vi "h.COMM.Write Command.vi"(6 "Request Option":T1, 8 "error in":errorcluster, 9 "Argument":string, 10 "Command":string, 11 "Connection ID":refnum<k5>) -> (0 "error out":errorcluster, 3 "Connection ID out":refnum<k5>)   [LabVIEW 2019, in "h.Library.lvlib"]
doc: "This vi sends a command and argument to a Hyperion instrument.\n\n<b>Connection ID</b> - is a network connection refnum that uniquely identifies the TCP connection\n<b>Command</b> - The command to execute\n<b>Request Options</b> - Option that controls how the command responds\n<b>error in</b> - describes error conditions that occur before this node runs. This input provides standard error functionality\n<b>Connection ID out</b> - Returns the same value as connection ID\n<b>error out</b> - contains error information. This output provides standard error out functionality."
uses:
  h.Library.lvlib
  CTL/h.COMM.RequestCommandOptions.ctl
panel:
  out "bytes written":i32
  # "Hyperion Write Command"
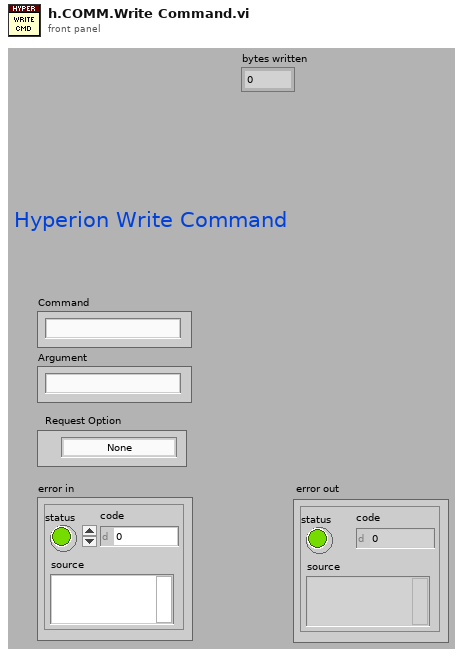
[diagram p1: front panel]
types:
  T1 = typedef "h.Library.lvlib/h.COMM.RequestCommandOptions.ctl" = enum8{"None", "Suppress Message", "Suppress Content", "Compress"}
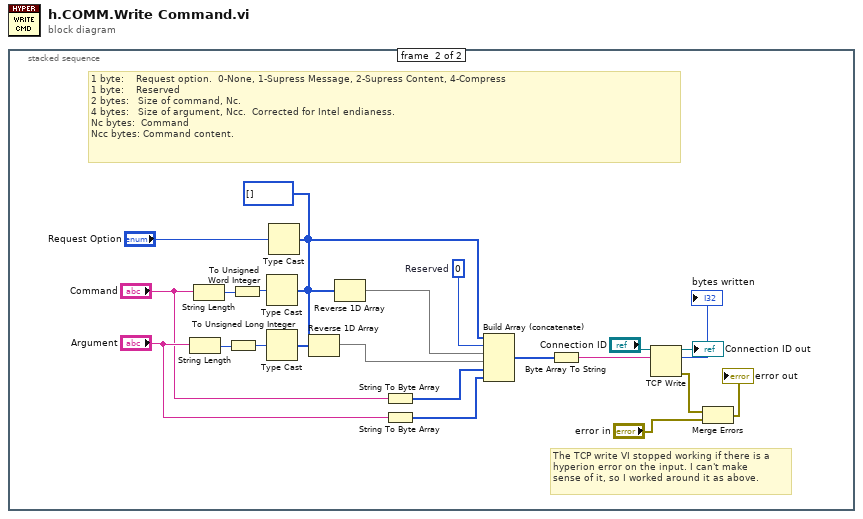
[diagram p0: block diagram]
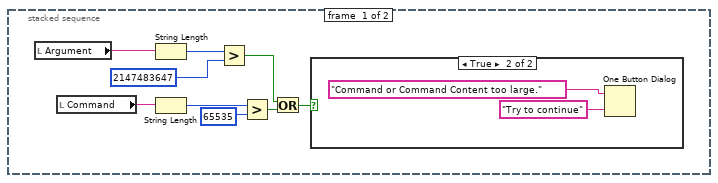
[diagram p2: hidden frame]
diagram:
  n1 = stacked-sequence {
    frame #0 {
      n2 = local read "Argument"() -> (w9:string)
      n3 = local read "Command"() -> (w8:string)
      n4 = String Length(string=w9) -> (length=w7:i32)
      n5 = String Length(string=w8) -> (length=w4:i32)
      n6 = Greater?(x=w7, y=2147483647) -> (0:w3:bool)
      n7 = Greater?(x=w4, y=65535) -> (0:w2:bool)
      n8 = Or(x=w3, y=w2) -> (x .or. y?=w1:bool)
      n9 = case shown="True" w1 {
        frame False {
        }
        frame True {
          n10 = One Button Dialog(message="Command or Command Content too large." ("[error source] (\" \")"), button name ("OK")="Try to continue") -> ()  [unwired: 1 out]
        }
      }
    }
    frame #1 {
      w22 = u8 0  # Reserved
      w16 = u8[] []
      # "The TCP write VI stopped working if there is a\nhyperion error on the input. I can't make\nsense of it, so I worked around it as above."
      # "1 byte:    Request option.  0-None, 1-Supress Message, 2-Supress Content, 4-Compress\n1 byte:    Reserved\n2 bytes:   Size of command, Nc.\n4 bytes:   Size of argument, Ncc.  Corrected for Intel endianess.\nNc bytes:  Command\nNcc bytes: Command content."
      n11 = String Length(string="Argument") -> (length=w32:i32)
      n12 = String Length(string="Command") -> (length=w33:i32)
      n13 = To Unsigned Long Integer(number=w32) -> (unsigned 32bit integer=w31:u32)
      n14 = To Unsigned Word Integer(number=w33) -> (unsigned 16bit integer=w21:u16)
      n15 = Type Cast(type=w16, x=w21) -> (*(type *) &x=w18:u8[])
      n16 = Type Cast(type=w16, x=w31) -> (*(type *) &x=w30:u8[])
      n17 = Type Cast(type=w16, x="Request Option") -> (*(type *) &x=w20:u8[])
      n18 = Reverse 1D Array(array=w30) -> (reversed array=w19:u8[])
      n19 = Reverse 1D Array(array=w18) -> (reversed array=w17:u8[])
      n20 = String To Byte Array(string="Command") -> (unsigned byte array=w26:u8[])
      n21 = String To Byte Array(string="Argument") -> (unsigned byte array=w27:u8[])
      n22 = Build Array (concatenate)(w20, w22, w17, w19, w26, w27) -> (w25:u8[])
      n23 = Byte Array To String(unsigned byte array=w25) -> (string=w24:string)
      n24 = TCP Write(connection ID="Connection ID", data in=w24) -> (connection ID out=→"Connection ID out":refnum<k5>, bytes written=→"bytes written":i32, error out=w14:errorcluster)  [unwired: 2 in]
      n25 = Merge Errors(w14, "error in") -> (→"error out":errorcluster)
    }
  }
